vi "Auto_Layup.vi"() -> (0 "Roller Commands":T4, 1 "Tipper Command Inputs":T3, 2 "Turret Command Inputs":T6, 3 "Conveyor Command Inputs":T1, 4 "Flywheel Commands":T5, 5 "Drive Command Inputs":T2)   [LabVIEW 2012]
uses:
  Turret/Inputs_Commands_Turret.ctl
  Flywheel/Input_Commands_Flywheel.ctl
  Roller/Input_Commands_Roller.ctl
  Bridge Tipper/Inputs_Tipper.ctl
  tankdrive/Input_Commands_Drive.ctl
  Conveyor/Input_Command_Conveyor.ctl
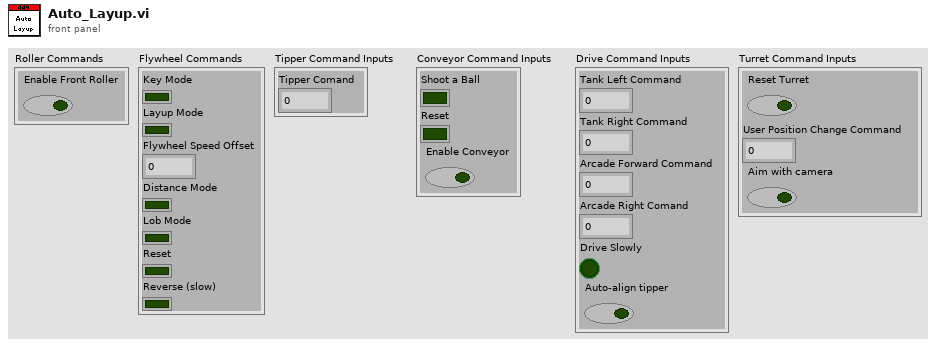
[diagram p1: front panel]
types:
  T1 = typedef "Input_Command_Conveyor.ctl" = cluster{"Shoot a Ball":bool, "Reset":bool, "Enable Conveyor":bool}
  T2 = typedef "Input_Commands_Drive.ctl" = cluster{"Tank Left Command":dbl, "Tank Right Command":dbl, "Arcade Forward Command":dbl, "Arcade Right Comand":dbl, "Drive Slowly":bool, "Auto-align tipper":bool}
  T3 = typedef "Inputs_Tipper.ctl" = cluster{"Tipper Comand":dbl}
  T4 = typedef "Input_Commands_Roller.ctl" = cluster{"Enable Front Roller":bool}
  T5 = typedef "Input_Commands_Flywheel.ctl" = cluster{"Key Mode":bool, "Layup Mode":bool, "Flywheel Speed Offset":dbl, "Distance Mode":bool, "Lob Mode":bool, "Reset":bool, "Reverse (slow)":bool}
  T6 = typedef "Inputs_Commands_Turret.ctl" = cluster{"Reset Turret":bool, "User Position Change Command":dbl, "Aim with camera":bool}
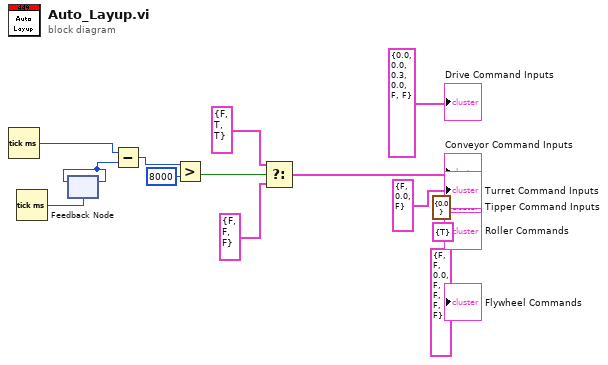
[diagram p0: block diagram]
diagram:
  n1 = Tick Count (ms)() -> (millisecond timer value=w2:u32)
  n2 = Tick Count (ms)() -> (millisecond timer value=w1:u32)
  n3 = feedback #1(w1) -> (w3:u32)
  n4 = feedback-in #1(w3) -> ()
  n5 = Subtract(x=w2, y=w3) -> (x-y=w4:u32)
  n6 = Greater?(x=w4, y=u32 8000) -> (0:w6:bool)
  n7 = Select(t=T1 {"Shoot a Ball"=FALSE, "Reset"=TRUE, "Enable Conveyor"=TRUE} ("Conveyor Command Inputs"), s=w6, f=T1 {"Shoot a Ball"=FALSE, "Reset"=FALSE, "Enable Conveyor"=FALSE} ("Conveyor Command Inputs")) -> (s? t:f=→"Conveyor Command Inputs":T1)
  "Turret Command Inputs" <- T6 {"Reset Turret"=FALSE, "User Position Change Command"=0.0, "Aim with camera"=FALSE} ("Turret Command Inputs")
  "Flywheel Commands" <- T5 {"Key Mode"=FALSE, "Layup Mode"=FALSE, "Flywheel Speed Offset"=0.0, "Distance Mode"=FALSE, "Lob Mode"=FALSE, "Reset"=FALSE, "Reverse (slow)"=FALSE} ("Flywheel Commands")
  "Roller Commands" <- T4 {"Enable Front Roller"=TRUE} ("Roller Commands")
  "Tipper Command Inputs" <- T3 {"Tipper Comand"=0.0} ("Tipper Command Inputs")
  "Drive Command Inputs" <- T2 {"Tank Left Command"=0.0, "Tank Right Command"=0.0, "Arcade Forward Command"=0.3, "Arcade Right Comand"=0.0, "Drive Slowly"=FALSE, "Auto-align tipper"=FALSE} ("Drive Command Inputs")
